vi "FPGA Server (9636).vi"() -> ()   [LabVIEW 2015]
doc: "This is the FPGA server for the sbRIO for the open-path cavity ring down."
uses:
  <vilib>/eio/EIONode/EIONode.xnode
  <vilib>/rvi/eio/common/nirviEmuTemplateMethod_errors.vi
  <vilib>/rvi/DataTransferAndStorage/Container/XNode/niFpgaContainer.xnode
  <vilib>/Platform/TimedLoop/XDataNode/XDataNode.xnode
  <vilib>/Platform/TimedLoop/XDataNode/nitl_modes.ctl
  <vilib>/Platform/TimedLoop/XDataNode/XDNodeRunTimeDep.lvlib
  <vilib>/Platform/TimedLoop/XDataNode/wakeup.ctl
  <vilib>/Platform/TimedLoop/XDataNode/timing_clust.ctl
  <vilib>/rvi/Memory/Memory_Emulation/nirvimemoryFastEmulation.vi
  <vilib>/rvi/Memory/Memory_Emulation/nirvimemoryEmulation.vi
  <vilib>/rvi/FXPMathLib/FxpMul/XNode/nifxpmath_Multiplier.xnode
  <vilib>/rvi/FXPMathLib/sim/FxpSim.dll
  <vilib>/rvi/interface/RandomDataEmulation/nirviRandomDataFpgaReadWriteTemplate.vi
  <vilib>/rvi/FXPMathLib/FxpDiv/XNode/nifxpmath_Div.xnode
  <vilib>/rvi/FXPMathLib/FxpDiv/simVIs/DllFxpDivTemp_sub.vi
  <vilib>/rvi/FXPMathLib/FxpDiv/subVIs/nifxpmath_Div_SimConfig.ctl
  Rate.ctl
panel:
  out "CollectData":bool
  in  "max":i32
  in  "InvertLaser?":bool
  in  "LaserOff (us)":u32
  in  "Reverse?":bool
  out "ShipError":bool
  out "EncodeLoop":bool
  out "LaserLoop":bool
  out "ShipLoop":bool
  out "DataLoop":bool
  out "Delay Ticks":u32
  in  "Delay (us)":u16
  out "RequestLaser":bool
  out "Sample Ticks":u32
  in  "Pause Digitizer":bool
  in  "Sample Time (us)":u16
  in  "Rate":T1=3 items=["1 MHz"=20, "2 MHz"=10, "2.5 MHz"=8, "5 MHz"=4, "10 MHz"=2, "20MHz"=1]
  out "LaserOFF?":bool
  in  "Cylce (ticks)":u32=40000
  out "DataRead":bool
  out "dataready":bool
  out "NewData":u16
  out "NumElements":u32
  in  "Stop":bool
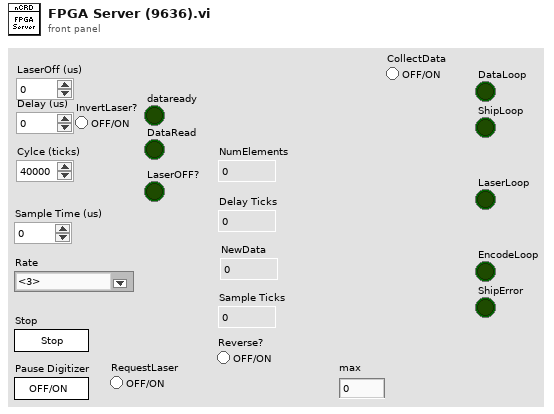
[diagram p1: front panel]
types:
  T1 = typedef "Rate.ctl" = u8
  T2 = cluster{"fixed-point type":fxp<+/-,64,64>, "x+y":fxp<+/-,64,64>, "x+y":fxp<+/-,64,64>, "x+y":fxp<+/-,64,64>, "x+y":fxp<+/-,64,64>, "x+y":fxp<+/-,64,64>, "x+y":fxp<+/-,64,64>}
  T3 = typedef "XDNodeRunTimeDep.lvlib/timing_clust.ctl" = cluster{"Expected End [f-1]":u64, "Actual End [f-1]":u64, "Finished Late? [f-1]":bool, "Expected End [i-1]":u64, "Actual End [i-1]":u64, "Finished Late? [i-1]":bool, "Expected Start [i]":u64, "Actual Start [i]":u64, "Expected Start [f]":u64, "Actual Start [f]":u64, "Source Name":string, "Structure Name":string, "Period":i64, "Deadline":i64, "Offset":i64, "Start":i64, "Priority":i32, "Timeout":i32, "Mode":T4, "Wakeup Reason":T5, "Error":errorcluster, "Source Type":string, "Secondary Source Type":string, "Global End Time":u64, "Global Start Time":u64, "Frame Duration":u64, "Iteration Duration":u64, "Assigned CPU":i32, "I/O Scan Engine Mode":u32}
  T4 = typedef "XDNodeRunTimeDep.lvlib/nitl_modes.ctl" = enum32{"No Change", "Process missed periods, maintain original phase", "Discard missed periods, maintain original phase", "Process missed periods, ignore original phase", "Discard missed periods, ignore original phase"}
  T5 = typedef "XDNodeRunTimeDep.lvlib/wakeup.ctl" = enum32{"Normal", "Aborted", "Asynchronous wakeup", "Timing source error", "Timed loop error", "Timeout"}
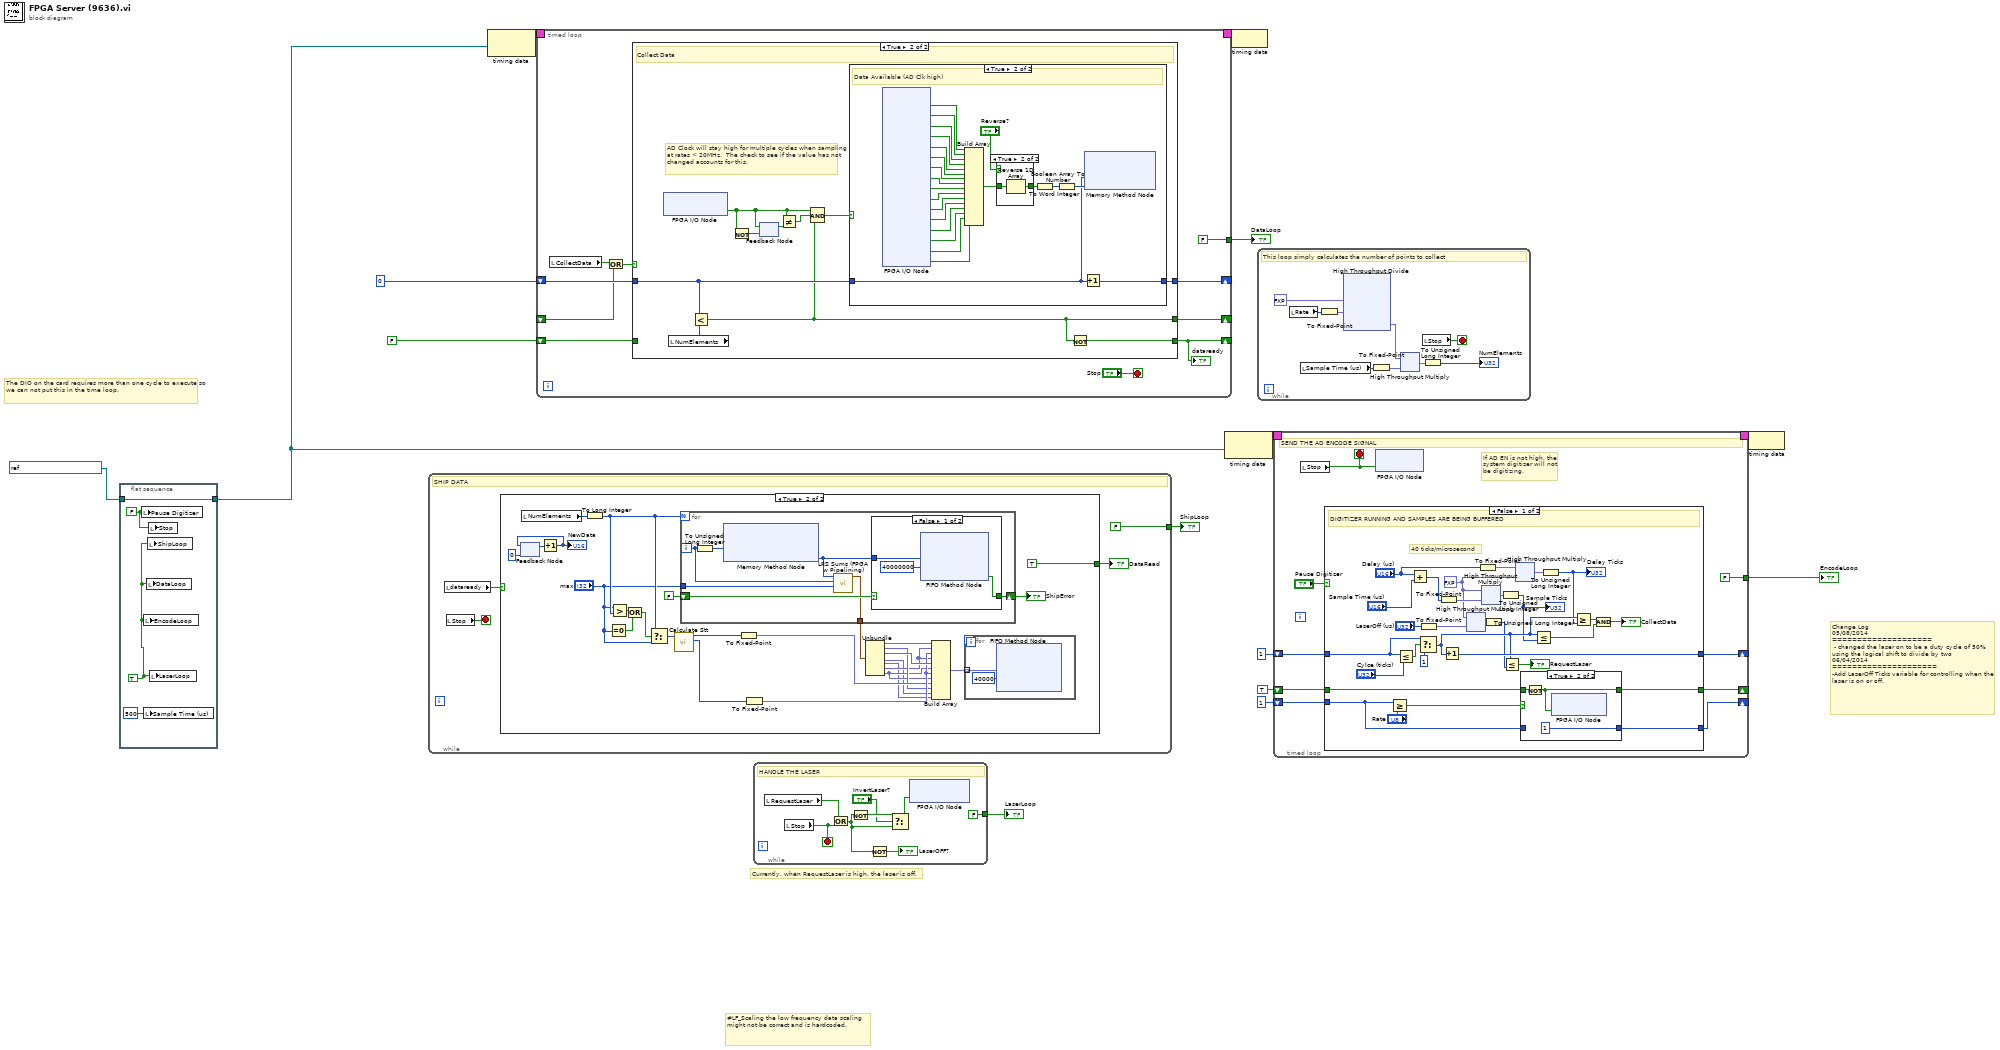
[diagram p0: block diagram]
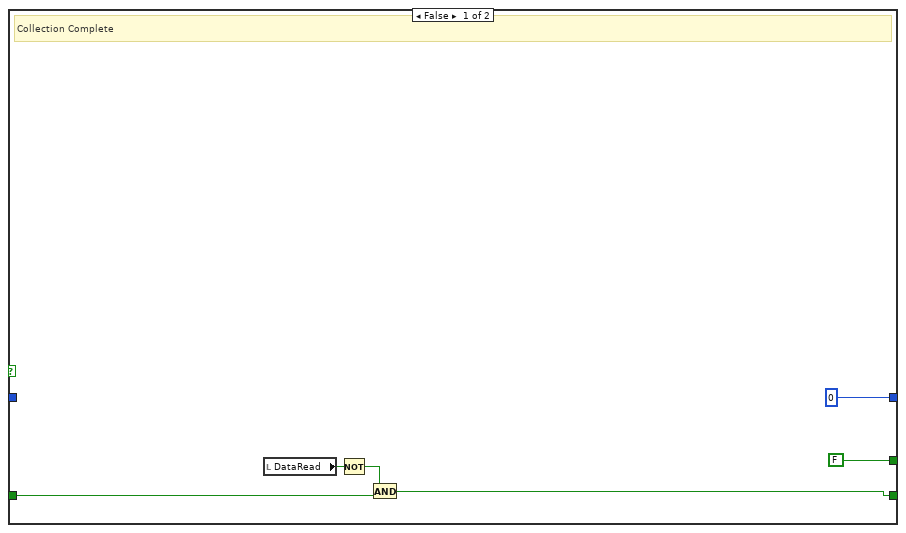
[diagram p2: hidden frame]
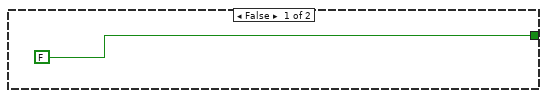
[diagram p5: hidden frame]
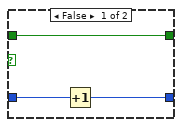
[diagram p7: hidden frame]
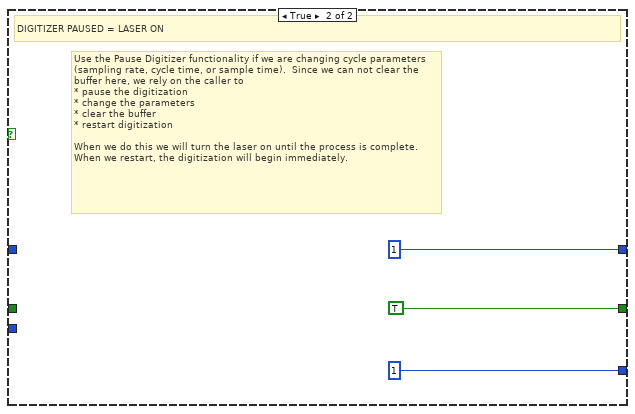
[diagram p8: hidden frame]
diagram:
  # "Change Log\n05/08/2014 \n====================\n - changed the laser on to be a duty cycle of 50% using the logical shift to divide by two\n06/04/2014\n=====================\n-Add LaserOff Ticks variable for controlling when the laser is on or off."
  # "Currently, when RequestLaser is high, the laser is off."
  # "#LF_Scaling the low frequency data scaling might not be correct and is hardcoded."
  # "The DIO on the card requires more than one cycle to execute so we can not put this in the time loop."
  n1 = flat-sequence {
    tunnel: refnum<k21> "40 MHz Onboard Clock" ("Source Name") -> [w19]
    tunnel: [w19] -> w1
    frame #0 {
      w17 = TRUE
      w18 = FALSE ("Pause Digitizer")
      n2 = local write "Pause Digitizer"(w18) -> ()
      n3 = local write "Sample Time (us)"(u16 500 ("Sample Time (us)")) -> ()
      n4 = local write "EncodeLoop"(w17) -> ()
      n5 = local write "DataLoop"(w17) -> ()
      n6 = local write "ShipLoop"(w17) -> ()
      n7 = local write "Stop"(w18) -> ()
      n8 = local write "LaserLoop"(w17) -> ()
    }
  }
  n9 = while {
    tunnel: [FALSE] -> w9
    stop <- w23 stop-if-true
    # "SHIP DATA"
    n10 = local read "dataready"() -> (w22:bool)
    n11 = local read "Stop"() -> (w23:bool)
    n12 = case shown="True" w22 {
      tunnel: [FALSE TRUE] -> w21
      frame False {
      }
      frame True {
        n13 = feedback #1(u16 0) -> (w48:u16)
        n14 = local read "NumElements"() -> (w44:u32)
        n15 = Increment(x=w48) -> (x+1=w49:u16)
        "NewData" <- w49
        n16 = feedback-in #1(w49) -> ()
        n17 = To Long Integer(number=w44) -> (32bit integer=w29:i32)
        n18 = Equal To 0?(x="max") -> (x = 0?=w26:bool)
        n19 = Greater?(x="max", y=w29) -> (0:w27:bool)
        n20 = Or(x=w27, y=w26) -> (x .or. y?=w25:bool)
        n21 = Select(t=w29, s=w25, f="max") -> (s? t:f=w43:i32)
        n22 = call "Calculate Stt.vi"("N"=w43) -> ("St"=w41:i64, "Stt"=w42:i64)  [unwired: 9 in]
        n23 = for {
          N: w29 -> [_]
          shift-right: [w56] -> w46
          shift-left: FALSE ("Timed Out?") -> [w55]
          tunnel: [w51] -> w36
          tunnel: "max" -> [w52]
          i -> [w54]
          n24 = To Unsigned Long Integer(number=w54) -> (unsigned 32bit integer=w57:u32)
          n25 = xnode ("Memory Method Node")("Address"=w57) -> ("Data"=w53:i16)  [unwired: 1 in, 1 out]
          n26 = call "LRS Sums (FPGA w Pipelining).vi"("max"=w52, "i"=w54, "DataIn"=w53) -> ("DataOut"=w51:T2)  [unwired: 8 in]
          n27 = case shown="False" w55 {
            selector: w55 -> [_ w61]
            tunnel: w53 -> [w60 _]
            tunnel: [w59 w61] -> w56
            frame False {
              n28 = xnode ("FIFO Method Node")("Element"=w60, "Timeout"=40000000) -> ("Timed Out?"=w59:bool)  [unwired: 1 in, 1 out]
            }
            frame True {
            }
          }
        }
        "ShipError" <- w46
        n29 = To Fixed-Point(number=w42) -> (fixed-point=w37:fxp<+/-,64,64>)  [unwired: 1 in]
        n30 = To Fixed-Point(number=w41) -> (fixed-point=w38:fxp<+/-,64,64>)  [unwired: 1 in]
        n31 = Unbundle(w36) -> ("fixed-point type"=w40:fxp<+/-,64,64>, "x+y"=w35:fxp<+/-,64,64>, "x+y"=w39:fxp<+/-,64,64>, "x+y"=w32:fxp<+/-,64,64>, "x+y"=w31:fxp<+/-,64,64>, "x+y"=w34:fxp<+/-,64,64>, "x+y"=w33:fxp<+/-,64,64>)
        n32 = Build Array(w40, w34, w38, w34, w39, w33, w38, w33, w37, w35, w32, w31) -> (w30:fxp<+/-,64,64>[])
        n33 = for {
          tunnel: w30 -> [w63] mode=indexing
          n34 = xnode ("FIFO Method Node")("Element"=w63, "Timeout"=40000) -> ()  [unwired: 1 in, 2 out]
        }
      }
    }
    "DataRead" <- w21
  }
  "ShipLoop" <- w9
  n35 = node-c288(w1) -> (w6:T3)
  n36 = timed-loop {
    timing: w6 -> [_]
    timing-out: [_] -> w5
    shift-right: [w71] -> _
    shift-left: u32 0 -> [w70]
    shift-right: [w69] -> _
    shift-left: _ -> [w68]
    shift-right: [w66] -> _
    shift-left: FALSE -> [w65]
    tunnel: [FALSE] -> w2
    stop <- "Stop" stop-if-true
    n37 = local read "CollectData"() -> (w73:bool)
    n38 = Or(x=w73, y=w68) -> (x .or. y?=w72:bool)
    n39 = case shown="True" w72 {
      tunnel: [u32 0 w85] -> w71
      tunnel: w70 -> [_ w86]
      tunnel: [FALSE w81] -> w69
      tunnel: [w74 w80] -> w66
      tunnel: w65 -> [w75 _]
      frame False {
        # "Collection Complete"
        n40 = local read "DataRead"() -> (w77:bool)
        n41 = Not(x=w77) -> (.not. x?=w76:bool)
        n42 = And(x=w76, y=w75) -> (x .and. y?=w74:bool)
      }
      frame True {
        # "AD Clock will stay high for multiple cycles when sampling at rates < 20MHz.  The check to see if the value has not changed accounts for this."
        # "Collect Data"
        n43 = xnode "FPGA I/O Node"() -> ("AD Clock +"=w83:bool)  [unwired: 1 in, 1 out]
        n44 = local read "NumElements"() -> (w89:u32)
        n45 = Less?(x=w86, y=w89) -> (x < y?=w81:bool)
        n46 = Not(x=w83) -> (.not. x?=w87:bool)
        n47 = feedback #2(w87) -> (w88:bool)
        n48 = feedback-in #2(w83) -> ()
        n49 = Not Equal?(x=w83, y=w88) -> (x != y?=w84:bool)
        n50 = Compound Arithmetic op=AND(w83, w84, w81) -> (w82:bool)
        n51 = case shown="True" w82 {
          tunnel: w86 -> [w90 w92]
          tunnel: [w90 w93] -> w85
          frame False {
            # "Waiting (Clk previously high or currently low)"
          }
          frame True {
            # "Data Available (AD Clk high)"
            n52 = xnode "FPGA I/O Node"() -> ("AD0"=w94:bool, "AD1"=w95:bool, "AD2"=w96:bool, "AD3"=w97:bool, "AD4"=w98:bool, "AD5"=w99:bool, "AD6"=w100:bool, "AD7"=w101:bool, "AD8"=w102:bool, "AD9"=w103:bool, "AD10"=w104:bool, "AD11"=w105:bool, "AD12"=w106:bool, "AD13"=w107:bool, "AD14"=w108:bool, "AD15"=w109:bool)  [unwired: 16 in, 16 out]
            n53 = Build Array(w94, w95, w96, w97, w98, w99, w100, w101, w102, w103, w104, w105, w106, w107, w108, w109) -> (w112:bool[])
            n54 = case shown="True" "Reverse?" {
              tunnel: w112 -> [w114 w116]
              tunnel: [w114 w115] -> w113
              frame False {
              }
              frame True {
                n55 = Reverse 1D Array(array=w116) -> (reversed array=w115:bool[])
              }
            }
            n56 = Boolean Array To Number(Boolean array=w113) -> (number=w110:u16)
            n57 = To Word Integer(number=w110) -> (16bit integer=w111:i16)
            n58 = Increment(x=w92) -> (x+1=w93:u32)
            n59 = xnode ("Memory Method Node")("Address"=w92, "Data"=w111) -> ()  [unwired: 1 in, 1 out]
          }
        }
        n60 = Not(x=w81) -> (.not. x?=w80:bool)
      }
    }
    "dataready" <- w66
  }
  "DataLoop" <- w2
  n61 = while {
    tunnel: [FALSE] -> w8
    stop <- w125 stop-if-true
    # "HANDLE THE LASER"
    n62 = local read "RequestLaser"() -> (w126:bool)
    n63 = local read "Stop"() -> (w125:bool)
    n64 = Or(x=w126, y=w125) -> (x .or. y?=w120:bool)
    n65 = Not(x=w120) -> (.not. x?=w122:bool)
    n66 = Not(x=w120) -> (.not. x?=→"LaserOFF?":bool)
    n67 = Select(t=w122, s="InvertLaser?", f=w120) -> (s? t:f=w121:bool)
    n68 = xnode "FPGA I/O Node"("Laser Mod"=w121) -> ()  [unwired: 1 in, 1 out]
  }
  "LaserLoop" <- w8
  n69 = node-c288(w1) -> (w15:T3)
  n70 = node-c288(w5) -> ()
  n71 = while {
    stop <- w135 stop-if-true
    # "This loop simply calculates the number of points to collect"
    n72 = local read "Rate"() -> (w131:T1)
    n73 = local read "Sample Time (us)"() -> (w134:u16)
    n74 = To Fixed-Point(number=w131) -> (fixed-point=w130:fxp<+,8,8>)  [unwired: 1 in]
    n75 = xnode "High Throughput Divide"("x"=fxp<+,8,8> 20.0 ("Sample Time (us) 2"), "y"=w130) -> ("x/y"=w129:fxp<+,16,8>)
    n76 = To Fixed-Point(number=w134) -> (fixed-point=w133:fxp<+,16,16>)  [unwired: 1 in]
    n77 = xnode ("High Throughput Multiply")("x"=w129, "y"=w133) -> ("x*y"=w128:fxp<+,32,32>)
    n78 = local read "Stop"() -> (w135:bool)
    n79 = To Unsigned Long Integer(number=w128) -> (unsigned 32bit integer=→"NumElements":u32)
  }
  n80 = timed-loop {
    shift-right: [w167] -> _
    shift-left: TRUE -> [w168]
    timing: w15 -> [_]
    timing-out: [_] -> w14
    shift-right: [w169] -> _
    shift-left: u32 1 -> [w170]
    shift-right: [w166] -> _
    shift-left: u8 1 -> [w165]
    tunnel: [FALSE] -> w7
    stop <- w171 stop-if-true
    # "If AD EN is not high, the system digitizer will not be digitizing."
    # "SEND THE AD ENCODE SIGNAL"
    n81 = local read "Stop"() -> (w171:bool)
    n82 = case shown="False" "Pause Digitizer" {
      tunnel: w170 -> [w184 _]
      tunnel: [w199 u32 1] -> w169
      tunnel: w168 -> [w196 _]
      tunnel: [w195 TRUE ("Element")] -> w167
      tunnel: [w194 u8 1] -> w166
      tunnel: w165 -> [w193 _]
      frame False {
        w180 = fxp<+,8,8> 40.0 ("Sample Time (us) 2")
        # "40 ticks/microsecond"
        # "DIGITIZER RUNNING AND SAMPLES ARE BEING BUFFERED"
        n83 = Greater Or Equal?(x=w193, y="Rate") -> (x >= y?=w197:bool)
        n84 = Less Or Equal?(x=w184, y="Cylce (ticks)") -> (x <= y?=w201:bool)
        n85 = Add(x="Delay (us)", y="Sample Time (us)") -> (x+y=w190:u16)
        n86 = Select(t=w184, s=w201, f=u32 1) -> (s? t:f=w182:u32)
        n87 = To Fixed-Point(number="LaserOff (us)") -> (fixed-point=w178:fxp<+,32,32>)  [unwired: 1 in]
        n88 = To Fixed-Point(number=w190) -> (fixed-point=w191:fxp<+,16,16>)  [unwired: 1 in]
        n89 = Increment(x=w182) -> (x+1=w199:u32)
        n90 = xnode ("High Throughput Multiply")("x"=w180, "y"=w178) -> ("x*y"=w177:fxp<+,32,32>)
        n91 = To Fixed-Point(number="Delay (us)") -> (fixed-point=w187:fxp<+,16,16>)  [unwired: 1 in]
        n92 = xnode ("High Throughput Multiply")("x"=w180, "y"=w191) -> ("x*y"=w192:fxp<+,32,32>)
        n93 = To Unsigned Long Integer(number=w177) -> (unsigned 32bit integer=w176:u32)
        n94 = To Unsigned Long Integer(number=w192) -> (unsigned 32bit integer=w172:u32)
        "Sample Ticks" <- w172
        n95 = Less Or Equal?(x=w182, y=w176) -> (x <= y?=→"RequestLaser":bool)
        n96 = xnode ("High Throughput Multiply")("x"=w187, "y"=w180) -> ("x*y"=w186:fxp<+,32,32>)
        n97 = case shown="True" w197 {
          tunnel: w196 -> [w204 w207]
          tunnel: [w204 w206] -> w195
          tunnel: [w202 u8 1] -> w194
          tunnel: w193 -> [w203 _]
          frame False {
            n98 = Increment(x=w203) -> (x+1=w202:u8)
          }
          frame True {
            n99 = Not(x=w207) -> (.not. x?=w206:bool)
            n100 = xnode "FPGA I/O Node"("ENCODE"=w206) -> ()  [unwired: 1 in, 1 out]
          }
        }
        n101 = Less Or Equal?(x=w182, y=w172) -> (x <= y?=w189:bool)
        n102 = To Unsigned Long Integer(number=w186) -> (unsigned 32bit integer=w173:u32)
        "Delay Ticks" <- w173
        n103 = Greater Or Equal?(x=w182, y=w173) -> (x >= y?=w185:bool)
        n104 = And(x=w185, y=w189) -> (x .and. y?=→"CollectData":bool)
      }
      frame True {
        # "Use the Pause Digitizer functionality if we are changing cycle parameters (sampling rate, cycle time, or sample time).  Since we can not clear the buffer here, we rely on the caller to \n* pause the digitization\n* change the parameters\n* clear the buffer\n* restart digitization\n\nWhen we do this we will turn the laser on until the process is complete. When we restart, the digitization will begin immediately."
        # "DIGITIZER PAUSED = LASER ON"
      }
    }
    n105 = xnode "FPGA I/O Node"("AD EN"=w171) -> ()  [unwired: 1 in, 1 out]
  }
  "EncodeLoop" <- w7
  n106 = node-c288(w14) -> ()
